vi "DBServerSettings.vi"() -> (0 "OK Button 2":bool)   [LabVIEW 2025]
uses:
  <vilib>/Utility/config.llb/NI_LVConfig.lvlib
  <vilib>/Utility/config.llb/Read Key (String).vi
  <vilib>/Utility/config.llb/Write Key (String).vi
panel:
  in  "Cancel Button":bool
  in  "OK Button":bool
  in  "Password":string
  in  "Username":string
  in  "Database":string
  in  "Server":string
  # "Database Server Settings"
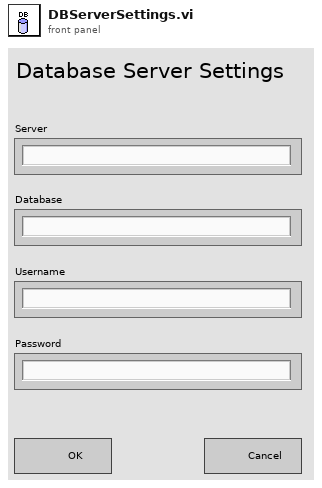
[diagram p1: front panel]
types:
  T1 = typedef "NI_LVConfig.lvlib/Config Data RefNum.ctl" = refnum<k1>
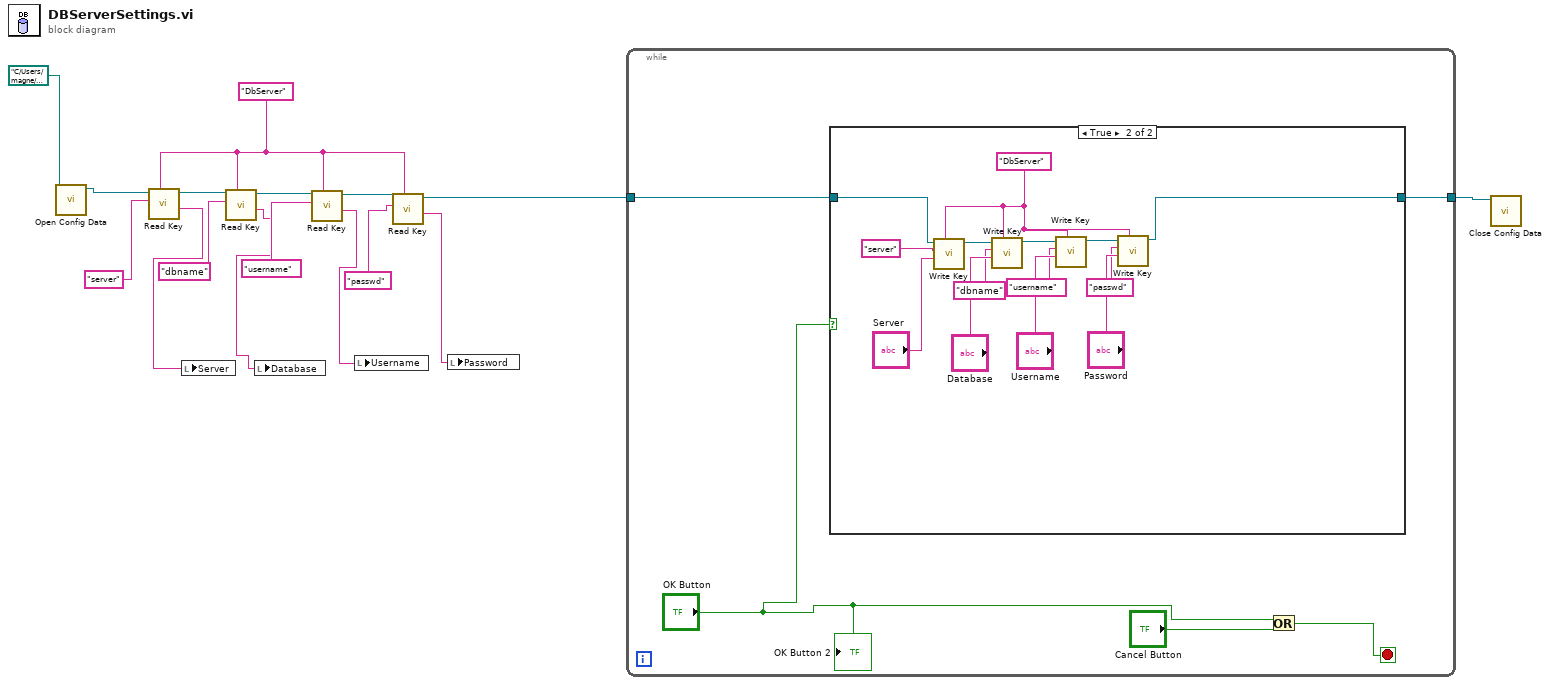
[diagram p0: block diagram]
diagram:
  w15 = "DbServer" ("section")
  n1 = call <vilib>:"Open Config Data.vi"("configuration file path"=path "C:/Users/magne/OneDrive/Dokumenter/Skole/IIA2017-1 26V Industrial Information Technology/Assignments/SCADA Assignment/02 Files/Task 3/settings.ini") -> ("refnum"=w9:T1)  [unwired: 8 in, 2 out]
  n2 = call-poly <vilib>:"Read Key.vi"("section"=w15, "key"="server", "refnum"=w9) -> ("value"=w6:string, "refnum out"=w10:T1)  [unwired: 5 in, 2 out]
  n3 = local write "Server"(w6) -> ()
  n4 = call-poly <vilib>:"Read Key.vi"("section"=w15, "key"="dbname", "refnum"=w10) -> ("value"=w5:string, "refnum out"=w8:T1)  [unwired: 5 in, 2 out]
  n5 = local write "Database"(w5) -> ()
  n6 = call-poly <vilib>:"Read Key.vi"("section"=w15, "key"="username", "refnum"=w8) -> ("value"=w4:string, "refnum out"=w7:T1)  [unwired: 5 in, 2 out]
  n7 = local write "Username"(w4) -> ()
  n8 = call-poly <vilib>:"Read Key.vi"("section"=w15, "key"="passwd", "refnum"=w7) -> ("value"=w3:string, "refnum out"=w1:T1)  [unwired: 5 in, 2 out]
  n9 = local write "Password"(w3) -> ()
  n10 = while {
    tunnel: [w18] -> w2
    tunnel: w1 -> [w17]
    stop <- w20 stop-if-true
    n11 = case shown="True" "OK Button" {
      tunnel: [w22 w29] -> w18
      tunnel: w17 -> [w22 w28]
      frame False {
      }
      frame True {
        w27 = "DbServer" ("section")
        n12 = call-poly <vilib>:"Write Key.vi"("section"=w27, "value"="Server", "key"="server", "refnum"=w28) -> ("refnum out"=w32:T1)  [unwired: 5 in, 2 out]
        n13 = call-poly <vilib>:"Write Key.vi"("section"=w27, "value"="Database", "key"="dbname", "refnum"=w32) -> ("refnum out"=w31:T1)  [unwired: 5 in, 2 out]
        n14 = call-poly <vilib>:"Write Key.vi"("section"=w27, "value"="Username", "key"="username", "refnum"=w31) -> ("refnum out"=w30:T1)  [unwired: 5 in, 2 out]
        n15 = call-poly <vilib>:"Write Key.vi"("section"=w27, "value"="Password", "key"="passwd", "refnum"=w30) -> ("refnum out"=w29:T1)  [unwired: 5 in, 2 out]
      }
    }
    n16 = Or(x="OK Button", y="Cancel Button") -> (x .or. y?=w20:bool)
    "OK Button 2" <- "OK Button"
  }
  n17 = call <vilib>:"Close Config Data.vi"("refnum"=w2) -> ()  [unwired: 9 in, 2 out]
